vi "writeHealthAndStatusControl.vi"(8 "error in (no error)":errorcluster, 9 "Timeout":i32, 10 "Data":u64[](array[numeric]), 11 "FPGA in":refnum<class "FPGA.lvclass">) -> (0 "error out":errorcluster, 2 "ElementsRemaining":u32, 3 "FPGA out":refnum<class "FPGA.lvclass">)   [LabVIEW 2016, in "FPGA.lvclass"]
uses:
  FPGA.lvclass
  FPGA.lvclass/FPGA.ctl
  <vilib>/Utility/error.llb/Error Cluster From Error Code.vi
  <vilib>/rvi/errors/niLvFpgaAdjustHostInterfaceError.vi
  <vilib>/rvi/interface/nirviMethod/nirviMethod.xnode
  <vilib>/FPGAPlugInAG/Dynamic/niLvFpga_WriteFifo_Dynamic.vi
  <vilib>/rvi/errors/niLvFpgaMergeErrorWithErrorCode.vi
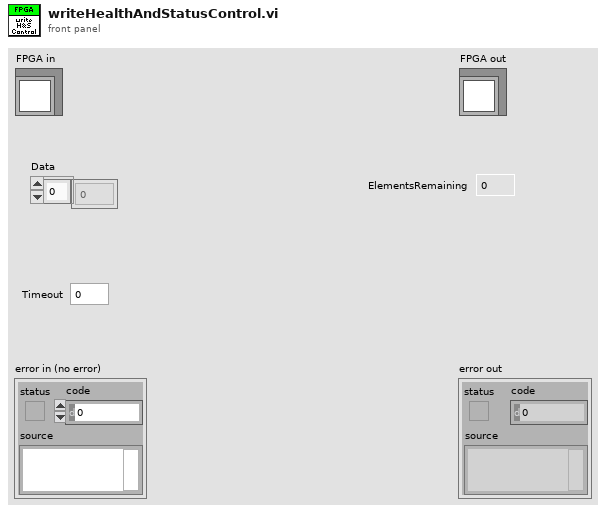
[diagram p1: front panel]
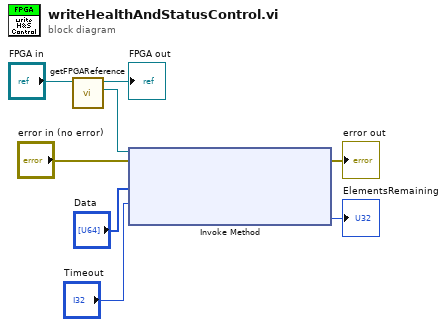
[diagram p0: block diagram]
diagram:
  n1 = call "getFPGAReference.vi"("FPGA in"="FPGA in") -> ("FPGAReference"=w7:refnum<k20>, "FPGA out"=→"FPGA out":refnum<class "FPGA.lvclass">)  [unwired: 9 in]
  n2 = xnode "Invoke Method"("FPGA VI Reference In"=w7, "error in"="error in (no error)", "Data"="Data", "Timeout (ms)"="Timeout") -> ("error out"=→"error out":errorcluster, "Empty Elements Remaining"=→"ElementsRemaining":u32)  [unwired: 1 out]
